vi "Write_Instr.vi"(8 "error in (no error)":errorcluster caption="entrée d'erreur (pas d'erreur)", 11 "Class Multimeter Multimeter en entrée":refnum<class "Class Instrument Schielding_Box.lvclass">) -> (0 "error out":errorcluster caption="sortie d'erreur", 3 "Class Multimeter Multimeter en sortie":refnum<class "Class Instrument Schielding_Box.lvclass">)   [LabVIEW 2020, in "Library Instrument & Equipement.lvlib" / "Library Instruments.lvlib" / "Class Instrument Schielding_Box.lvclass"]
uses:
  Class Instrument Schielding_Box.lvclass
  Class Instrument Schielding_Box.lvclass/Class Instrument Schielding_Box.ctl
  Instrument (Default)/Class Instrument (Default).lvclass
  Shielding box/Class Shielding box (Default)/Class Shielding_ Box (Default).lvclass
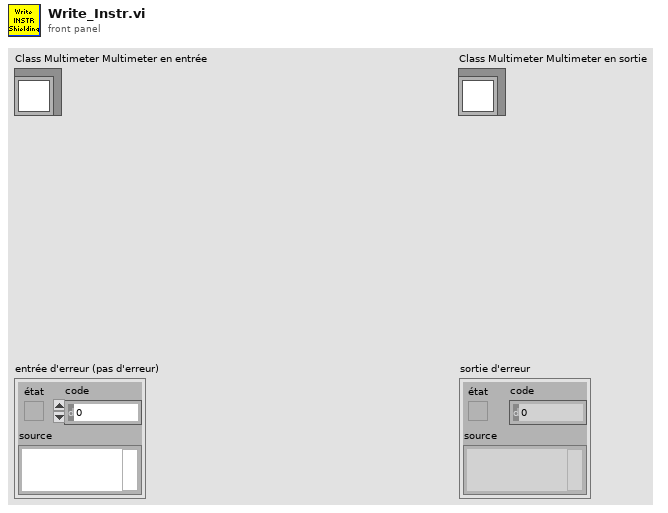
[diagram p1: front panel]
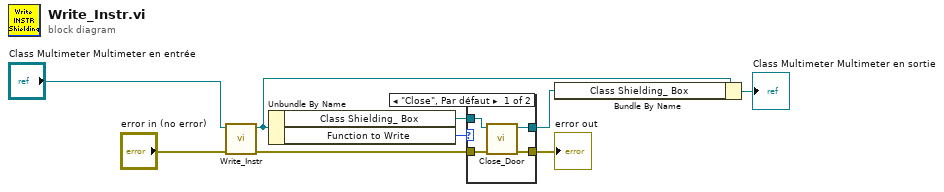
[diagram p0: block diagram]
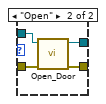
[diagram p2: hidden frame]
diagram:
  n1 = call-parent "Write_Instr.vi"("error in (no error)"="error in (no error)", "Class Multimeter (Default) en entrée"="Class Multimeter Multimeter en entrée") -> ("error out"=w2:errorcluster, "Class Multimeter (Default) en sortie"=w6:refnum<class "Class Instrument Schielding_Box.lvclass">)  [unwired: 8 in]
  n2 = Unbundle By Name(w6) -> ("Class Shielding_ Box"=w4:refnum<class "Class Shielding_ Box (Default).lvclass">, "Function to Write"=w5:enum16{"Close", "Open"})
  n3 = case shown="\"Close\", Par défaut" w5 {
    tunnel: w4 -> [w12 w17]
    tunnel: [w11 w16] -> w3
    tunnel: w2 -> [w13 w15]
    tunnel: [w10 w14] -> w1
    frame "Close", Default {
      n4 = call-dynamic "Close_Door.vi"("error in (no error)"=w13, "Class Shielding_ Box en entrée"=w12) -> ("error out"=w10:errorcluster, "Class Shielding_ Box en sortie"=w11:refnum<class "Class Shielding_ Box (Default).lvclass">)  [unwired: 8 in]
    }
    frame "Open" {
      n5 = call-dynamic "Open_Door.vi"("error in (no error)"=w15, "Class Shielding_ Box en entrée"=w17) -> ("error out"=w14:errorcluster, "Class Shielding_ Box en sortie"=w16:refnum<class "Class Shielding_ Box (Default).lvclass">)  [unwired: 8 in]
    }
  }
  "error out" <- w1
  n6 = Bundle By Name(cluster=w6, "Class Shielding_ Box"=w3) -> (→"Class Multimeter Multimeter en sortie":refnum<class "Class Instrument Schielding_Box.lvclass">)
